vi "main.vi"() -> ()   [LabVIEW 2026]
uses:
  <vilib>/Instr/_visa.llb/VISA Configure Serial Port (Instr).vi
panel:
  out "原始波形chart":dbl[](graph)
  out "原始波形graph":dbl[](graph)
  out "采样值数组":i16[](array[numeric])
  out "当前帧长度":i32
  out "状态显示":string
  in  "Button 2":bool
  in  "每帧点数":i32
  in  "Button":bool
  in  "采样率fs":dbl format="%#_13g"
  in  "baud rate 波特率":u32=9600
  in  "VISA resource name":refnum<visa-resource-name>
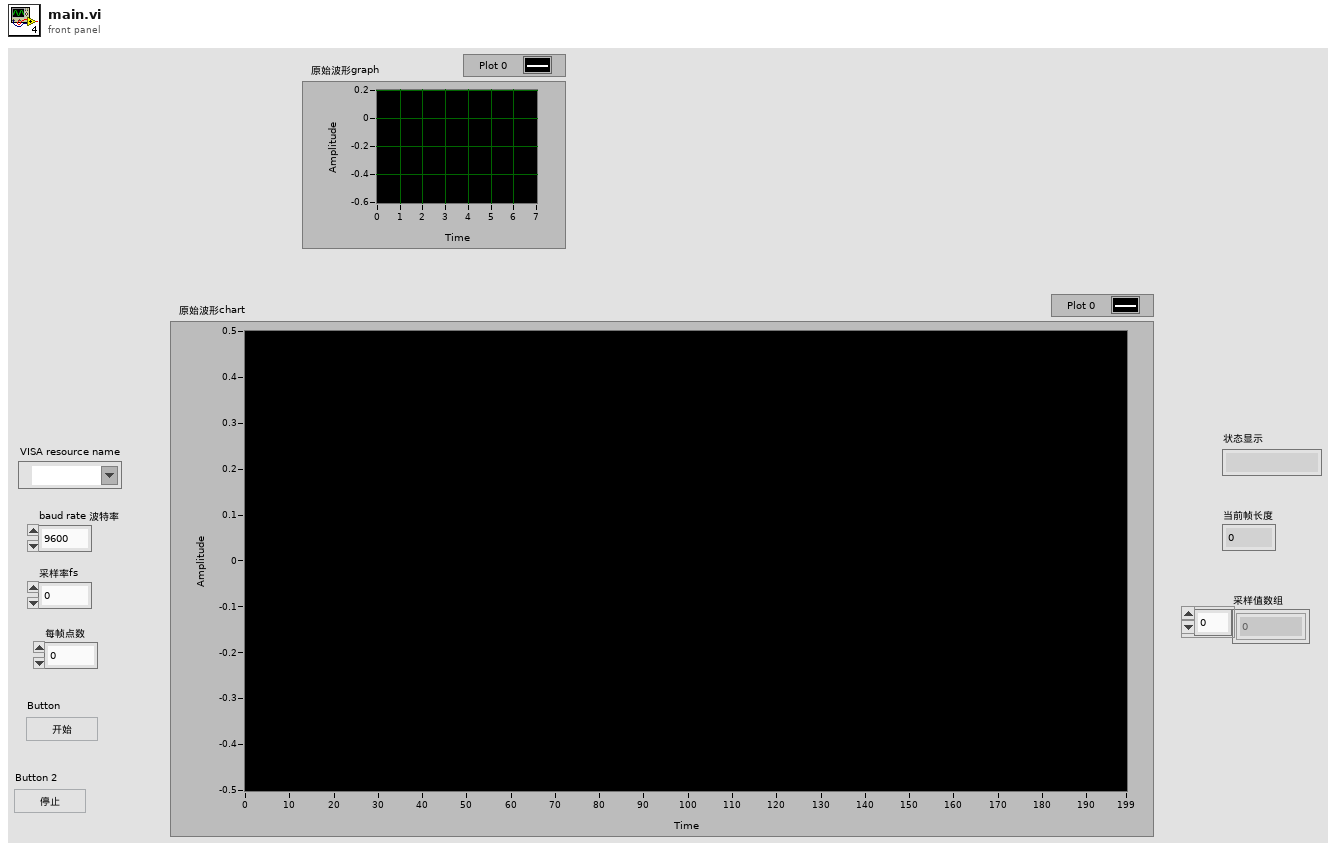
[diagram p1: front panel]
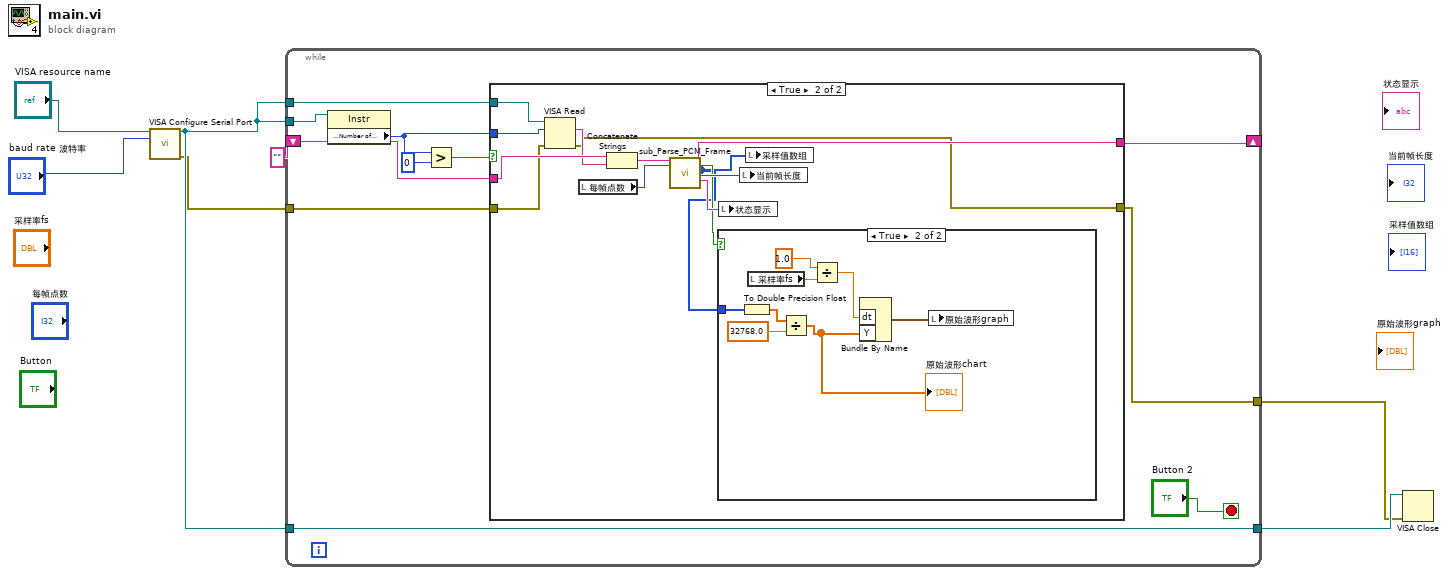
[diagram p0: block diagram]
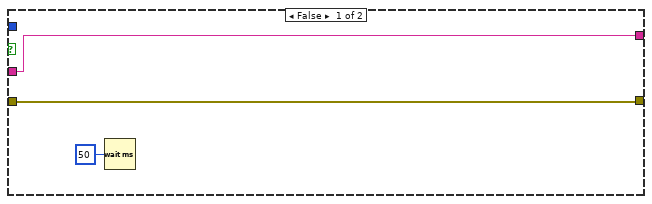
[diagram p2: hidden frame]
diagram:
  n1 = call-poly "VISA Configure Serial Port"("VISA resource name"="VISA resource name", "baud rate (9600)"="baud rate 波特率") -> ("VISA resource name out"=w4:refnum<visa-resource-name>, "error out"=w2:errorcluster)  [unwired: 12 in]
  n2 = while {
    shift-right: [w13] -> _
    shift-left: "" -> [w14]
    tunnel: w4 -> [w15]
    tunnel: w4 -> [w12]
    tunnel: w4 -> [w11]
    tunnel: [w11] -> w3
    tunnel: w2 -> [w10]
    tunnel: [w9] -> w1
    stop <- "Button 2" stop-if-true
    n3 = property class="Instr"(reference=w12) -> ("Serial Settings:Number of Bytes at Serial Port"=w16:u32)  [unwired: 1 in, 2 out]
    n4 = Greater?(x=w16, y=u32 0) -> (0:w17:bool)
    n5 = case shown="True" w17 {
      tunnel: w16 -> [_ w34]
      tunnel: w15 -> [_ w33]
      tunnel: w14 -> [w20 w32]
      tunnel: [w20 w26] -> w13
      tunnel: w10 -> [w19 w24]
      tunnel: [w19 w23] -> w9
      frame False {
        n6 = Wait (ms)(milliseconds to wait=u32 50) -> ()  [unwired: 1 out]
      }
      frame True {
        n7 = VISA Read(VISA resource name=w33, byte count=w34, error in (no error)=w24) -> (read buffer=w31:string, error out=w23:errorcluster)  [unwired: 2 out]
        n8 = local read "每帧点数"() -> (w29:i32)
        n9 = Concatenate Strings(w32, w31) -> (w30:string)
        n10 = call "sub_Parse_PCM_Frame.vi"("In Buffer"=w30, "每帧点数N"=w29) -> ("Out Buffer"=w26:string, "valid？"=w25:bool, "Samples  I16"=w22:i16[], "Frame Length"=w27:u32, "Parse Status"=w28:string)  [unwired: 13 in]
        n11 = case shown="True" w25 {
          tunnel: w22 -> [_ w42]
          frame False {
          }
          frame True {
            n12 = To Double Precision Float(number=w42) -> (double precision float=w41:dbl[])
            n13 = local read "采样率fs"() -> (w39:dbl)
            n14 = Divide(x=w41, y=32768.0) -> (x/y=w35:dbl[])
            "原始波形chart" <- w35
            n15 = Divide(x=1.0, y=w39) -> (x/y=w37:dbl)
            n16 = Bundle By Name("dt"=w37, "Y"=w35) -> (w36:waveform(dbl))  [unwired: 1 in]
            n17 = local write "原始波形graph"(w36) -> ()
          }
        }
        n18 = local write "状态显示"(w28) -> ()
        n19 = local write "当前帧长度"(w27) -> ()
        n20 = local write "采样值数组"(w22) -> ()
      }
    }
  }
  n21 = VISA Close(VISA resource name=w3, error in (no error)=w1) -> ()  [unwired: 1 out]
